vi "MultitaskExample.vi"() -> ()   [LabVIEW 2015]
uses:
  <vilib>/NI/cRIO Wfm/ChannelConfig.ctl
  <vilib>/FPGAPlugInAG/sbRIO-9607/niLvFpga_Open_sbRIO-9607.vi
  <vilib>/rvi/interface/common/dynamic/niFpgaDynamicAddResources.vi
  <vilib>/FPGAPlugInAG/Dynamic/niLvFpga_Reset_Dynamic.vi
  <vilib>/FPGAPlugInAG/Dynamic/niLvFpga_Run_Dynamic.vi
  ReadWaveform.vi
  Read2D.vi
  <vilib>/Utility/error.llb/Error Cluster From Error Code.vi
  <vilib>/rvi/errors/niLvFpgaAdjustHostInterfaceError.vi
  <vilib>/FPGAPlugInAG/Dynamic/niLvFpga_Close_Dynamic.vi
  <vilib>/rvi/interface/nirviOpenFPGA/nirviOpenFPGA.xnode
  FPGA Bitfiles/WaveformLibraryI_FPGATarget2_[FPGA]SARAcqMain_U+qOsuK4w1s.lvbitx
  <vilib>/rvi/interface/nirviMethod/nirviMethod.xnode
  <vilib>/rvi/interface/nirviReadWriteControl/nirviReadWriteControl.xnode
  <vilib>/rvi/interface/nirviCloseFPGA/nirviCloseFPGA.xnode
  <instrlib>/_niInstr/FIFO Register Bus/v1/Host/niInstr FIFO Register Bus v1 Host.lvclass
  WaveformTask.lvclass
  <vilib>/NI/cRIO Wfm/cRIO Wfm.lvlib
  NiFpgaLv.dll
  <vilib>/rvi/interface/Simulation/niFpgaSimulationCallBeginRW.vi
panel:
  in  "stop":bool
  in  "injectError0":errorcluster
  out "Data 4":waveform(sgl)[](graph)
  out "Data 3":sgl[][](graph)
  out "Data 2":sgl[][](graph)
  out "Data":waveform(sgl)[](graph)
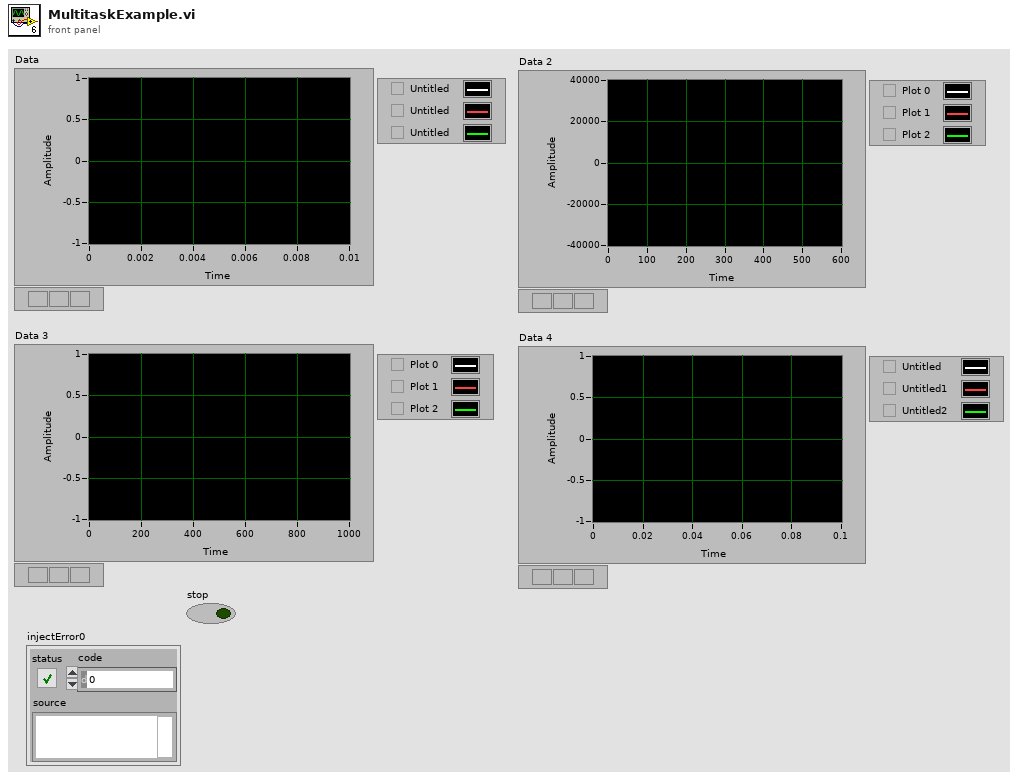
[diagram p1: front panel]
types:
  T1 = typedef "cRIO Wfm.lvlib/ChannelConfig.ctl" = cluster{"Channel Name":string, "Sensitivity mV_EU":dbl, "EU":string, "dB Ref EU":dbl}[]
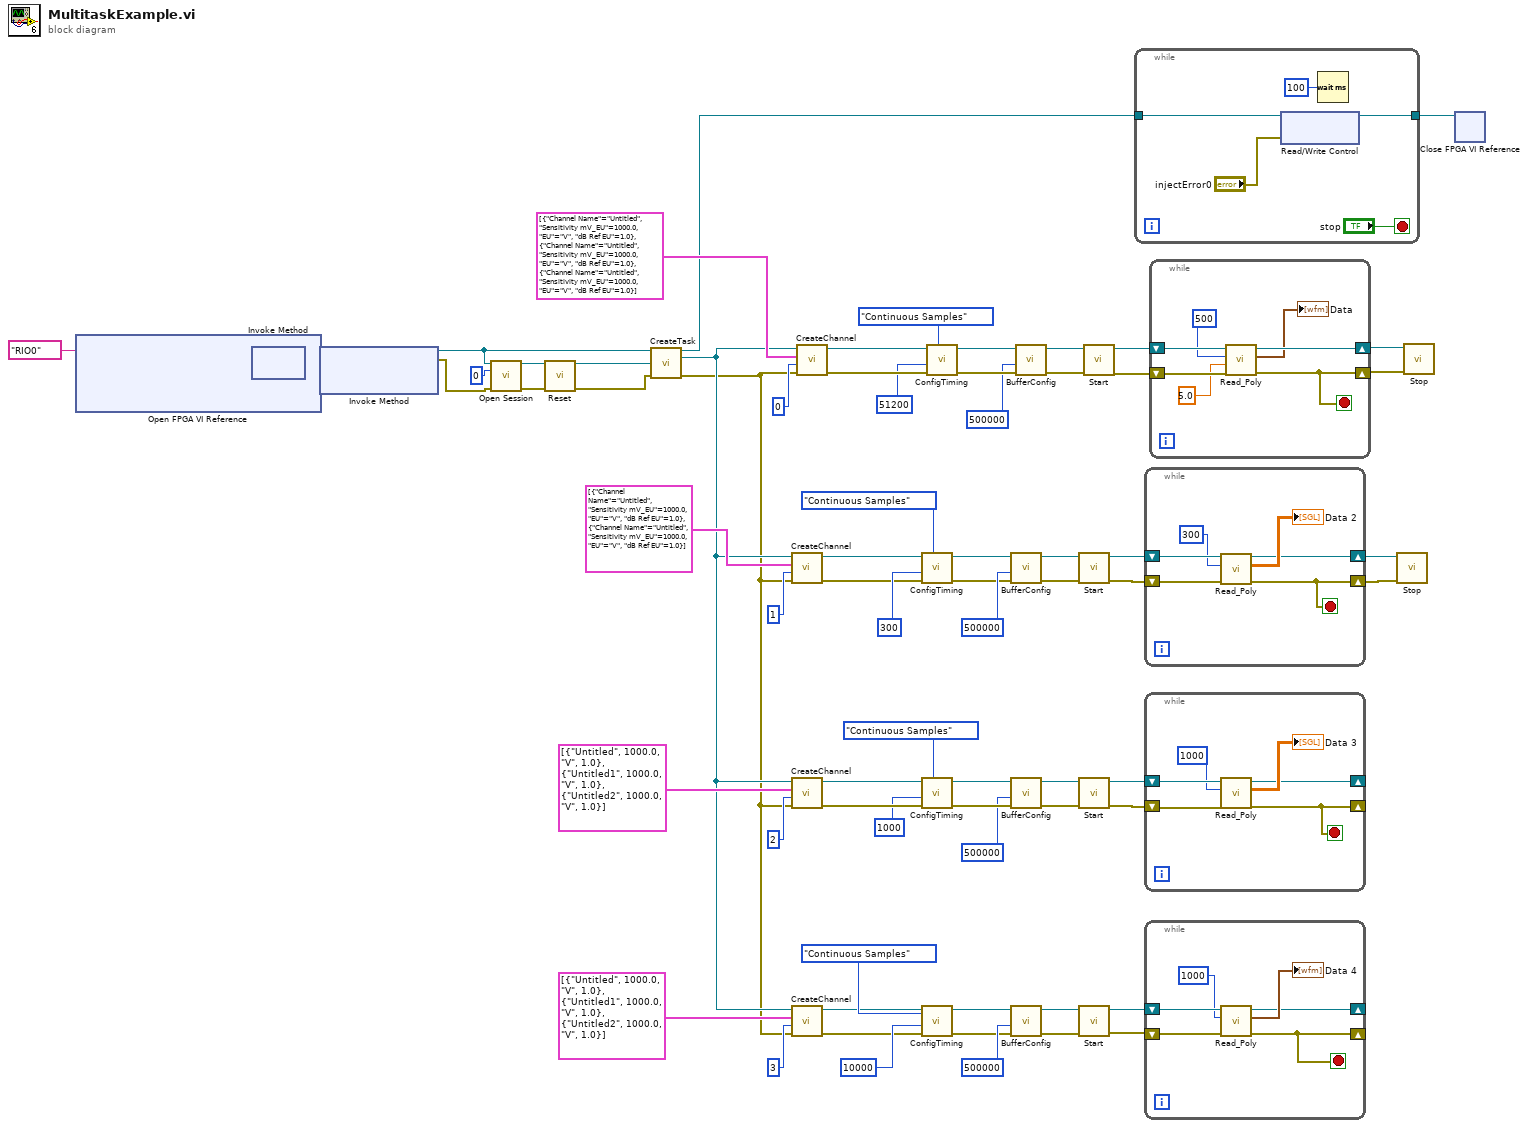
[diagram p0: block diagram]
diagram:
  n1 = xnode "Open FPGA VI Reference"("resource name"=tag "RIO0") -> ("FPGA VI Reference Out"=w59:refnum<k20>, "error out"=w58:errorcluster)  [unwired: 1 in]
  n2 = xnode "Invoke Method"("FPGA VI Reference In"=w59, "error in"=w58) -> ("FPGA VI Reference Out"=w57:refnum<k20>, "error out"=w56:errorcluster)
  n3 = xnode "Invoke Method"("FPGA VI Reference In"=w57, "error in"=w56) -> ("FPGA VI Reference Out"=w3:refnum<k20>, "error out"=w4:errorcluster)  [unwired: 1 in]
  n4 = call <instrlib>:"Open Session.vi"("fpga ref"=w3, "bus instance"=u32 0, "error in"=w4) -> ("session out"=w6:refnum<class "niInstr FIFO Register Bus v1 Host.lvclass">, "error out"=w7:errorcluster)  [unwired: 11 in]
  n5 = call-dynamic "Reset.vi"("session in"=w6, "error in"=w7) -> ("session out"=w2:refnum<class "niInstr FIFO Register Bus v1 Host.lvclass">, "error out"=w1:errorcluster)  [unwired: 12 in]
  n6 = call "CreateTask.vi"("FPGA Ref in"=w3, "session in"=w2, "error in"=w1) -> ("FPGA Ref out"=w41:refnum<k20>, "Task out"=w14:refnum<class "WaveformTask.lvclass">, "error out"=w13:errorcluster)  [unwired: 9 in, 1 out]
  n7 = call "CreateChannel.vi"("error in"=w13, "instance"=u8 1, "Channel Info"=T1 [{"Channel Name"="Untitled", "Sensitivity mV_EU"=1000.0, "EU"="V", "dB Ref EU"=1.0}, {"Channel Name"="Untitled", "Sensitivity mV_EU"=1000.0, "EU"="V", "dB Ref EU"=1.0}], "task in"=w14) -> ("error out"=w46:errorcluster, "Task out"=w42:refnum<class "WaveformTask.lvclass">)  [unwired: 6 in]
  n8 = call "CreateChannel.vi"("error in"=w13, "instance"=u8 2, "Channel Info"=T1 [{"Channel Name"="Untitled", "Sensitivity mV_EU"=1000.0, "EU"="V", "dB Ref EU"=1.0}, {"Channel Name"="Untitled1", "Sensitivity mV_EU"=1000.0, "EU"="V", "dB Ref EU"=1.0}, {"Channel Name"="Untitled2", "Sensitivity mV_EU"=1000.0, "EU"="V", "dB Ref EU"=1.0}], "task in"=w14) -> ("error out"=w38:errorcluster, "Task out"=w40:refnum<class "WaveformTask.lvclass">)  [unwired: 6 in]
  n9 = call "CreateChannel.vi"("error in"=w13, "instance"=u8 3, "Channel Info"=T1 [{"Channel Name"="Untitled", "Sensitivity mV_EU"=1000.0, "EU"="V", "dB Ref EU"=1.0}, {"Channel Name"="Untitled1", "Sensitivity mV_EU"=1000.0, "EU"="V", "dB Ref EU"=1.0}, {"Channel Name"="Untitled2", "Sensitivity mV_EU"=1000.0, "EU"="V", "dB Ref EU"=1.0}], "task in"=w14) -> ("error out"=w17:errorcluster, "Task out"=w15:refnum<class "WaveformTask.lvclass">)  [unwired: 6 in]
  n10 = call "CreateChannel.vi"("error in"=w13, "instance"=u8 0, "Channel Info"=T1 [{"Channel Name"="Untitled", "Sensitivity mV_EU"=1000.0, "EU"="V", "dB Ref EU"=1.0}, {"Channel Name"="Untitled", "Sensitivity mV_EU"=1000.0, "EU"="V", "dB Ref EU"=1.0}, {"Channel Name"="Untitled", "Sensitivity mV_EU"=1000.0, "EU"="V", "dB Ref EU"=1.0}], "task in"=w14) -> ("error out"=w69:errorcluster, "Task out"=w43:refnum<class "WaveformTask.lvclass">)  [unwired: 6 in]
  n11 = call "ConfigTiming.vi"("Sample Mode"=enum16{"Finite Samples", "Continuous Samples"}."Continuous Samples", "error in (no error)"=w46, "Sample Rate"=u32 300, "Task in"=w42) -> ("error out"=w50:errorcluster, "Task out"=w49:refnum<class "WaveformTask.lvclass">)  [unwired: 5 in, 1 out]
  n12 = call "ConfigTiming.vi"("Sample Mode"=enum16{"Finite Samples", "Continuous Samples"}."Continuous Samples", "error in (no error)"=w38, "Sample Rate"=u32 1000, "Task in"=w40) -> ("error out"=w34:errorcluster, "Task out"=w35:refnum<class "WaveformTask.lvclass">)  [unwired: 5 in, 1 out]
  n13 = call "ConfigTiming.vi"("Sample Mode"=enum16{"Finite Samples", "Continuous Samples"}."Continuous Samples", "error in (no error)"=w17, "Sample Rate"=u32 10000, "Task in"=w15) -> ("error out"=w21:errorcluster, "Task out"=w20:refnum<class "WaveformTask.lvclass">)  [unwired: 5 in, 1 out]
  n14 = call "ConfigTiming.vi"("Sample Mode"=enum16{"Finite Samples", "Continuous Samples"}."Continuous Samples", "error in (no error)"=w69, "Sample Rate"=u32 51200, "Task in"=w43) -> ("error out"=w65:errorcluster, "Task out"=w66:refnum<class "WaveformTask.lvclass">)  [unwired: 5 in, 1 out]
  n15 = call "BufferConfig.vi"("error in (no error)"=w50, "Buffer Size [Samps per Chan]"=500000, "WaveformTask in"=w49) -> ("error out"=w53:errorcluster, "WaveformTask out"=w52:refnum<class "WaveformTask.lvclass">)  [unwired: 6 in, 1 out]
  n16 = call "BufferConfig.vi"("error in (no error)"=w34, "Buffer Size [Samps per Chan]"=500000, "WaveformTask in"=w35) -> ("error out"=w31:errorcluster, "WaveformTask out"=w32:refnum<class "WaveformTask.lvclass">)  [unwired: 6 in, 1 out]
  n17 = call "BufferConfig.vi"("error in (no error)"=w21, "Buffer Size [Samps per Chan]"=500000, "WaveformTask in"=w20) -> ("error out"=w24:errorcluster, "WaveformTask out"=w23:refnum<class "WaveformTask.lvclass">)  [unwired: 6 in, 1 out]
  n18 = call "BufferConfig.vi"("error in (no error)"=w65, "Buffer Size [Samps per Chan]"=500000, "WaveformTask in"=w66) -> ("error out"=w62:errorcluster, "WaveformTask out"=w63:refnum<class "WaveformTask.lvclass">)  [unwired: 6 in, 1 out]
  n19 = call "Start.vi"("error in (no error)"=w53, "WaveformTask in"=w52) -> ("error out"=w55:errorcluster, "WaveformTask out"=w54:refnum<class "WaveformTask.lvclass">)  [unwired: 8 in]
  n20 = call "Start.vi"("error in (no error)"=w31, "WaveformTask in"=w32) -> ("error out"=w29:errorcluster, "WaveformTask out"=w30:refnum<class "WaveformTask.lvclass">)  [unwired: 8 in]
  n21 = call "Start.vi"("error in (no error)"=w24, "WaveformTask in"=w23) -> ("error out"=w26:errorcluster, "WaveformTask out"=w25:refnum<class "WaveformTask.lvclass">)  [unwired: 8 in]
  n22 = call "Start.vi"("error in (no error)"=w62, "WaveformTask in"=w63) -> ("error out"=w60:errorcluster, "WaveformTask out"=w61:refnum<class "WaveformTask.lvclass">)  [unwired: 8 in]
  n23 = while {
    tunnel: w41 -> [w75]
    tunnel: [w74] -> w8
    stop <- "stop" stop-if-true
    n24 = xnode "Read/Write Control"("FPGA VI Reference In"=w75, "injectError0"="injectError0") -> ("FPGA VI Reference Out"=w74:refnum<k20>)  [unwired: 1 in, 1 out]
    n25 = Wait (ms)(milliseconds to wait=u32 100) -> ()  [unwired: 1 out]
  }
  n26 = while {
    shift-right: [w78] -> w9
    shift-left: w55 -> [w82]
    shift-right: [w80] -> w10
    shift-left: w54 -> [w83]
    stop <- w78 stop-if-true
    n27 = call-poly "Read_Poly.vi"("error in"=w82, "Samps Read per Chan"=300, "Task in"=w83) -> ("error out"=w78:errorcluster, "Data"=→"Data 2":sgl[][], "Task out"=w80:refnum<class "WaveformTask.lvclass">)  [unwired: 5 in, 1 out]
  }
  n28 = while {
    shift-right: [w84] -> _
    shift-left: w29 -> [w88]
    shift-right: [w86] -> _
    shift-left: w30 -> [w89]
    stop <- w84 stop-if-true
    n29 = call-poly "Read_Poly.vi"("error in"=w88, "Samps Read per Chan"=1000, "Task in"=w89) -> ("error out"=w84:errorcluster, "Data"=→"Data 3":sgl[][], "Task out"=w86:refnum<class "WaveformTask.lvclass">)  [unwired: 5 in, 1 out]
  }
  n30 = while {
    shift-right: [w90] -> _
    shift-left: w26 -> [w94]
    shift-right: [w92] -> _
    shift-left: w25 -> [w95]
    stop <- w90 stop-if-true
    n31 = call-poly "Read_Poly.vi"("error in"=w94, "Samps Read per Chan"=1000, "Task in"=w95) -> ("error out"=w90:errorcluster, "Waveforms"=→"Data 4":waveform(sgl)[], "Task out"=w92:refnum<class "WaveformTask.lvclass">)  [unwired: 5 in, 1 out]
  }
  n32 = while {
    shift-right: [w96] -> w11
    shift-left: w60 -> [w101]
    shift-right: [w98] -> w12
    shift-left: w61 -> [w102]
    stop <- w96 stop-if-true
    n33 = call-poly "Read_Poly.vi"("error in"=w101, "Timeout (s)"=5.0, "Samps Read per Chan"=500, "Task in"=w102) -> ("error out"=w96:errorcluster, "Waveforms"=→"Data":waveform(sgl)[], "Task out"=w98:refnum<class "WaveformTask.lvclass">)  [unwired: 4 in, 1 out]
  }
  n34 = call "Stop.vi"("error in"=w9, "WaveformTask in"=w10) -> ()  [unwired: 8 in, 2 out]
  n35 = call "Stop.vi"("error in"=w11, "WaveformTask in"=w12) -> ()  [unwired: 8 in, 2 out]
  n36 = xnode "Close FPGA VI Reference"("FPGA VI Reference In"=w8) -> ()  [unwired: 1 in, 1 out]
